vi "set_gate_parameters.vi"(4 "repetitions":i64, 5 "pulse duration (iterations)":i64, 6 "offset duration (iterations)":i64, 7 "gate no.":i32, 8 "error in (no error)":errorcluster, 9 "low phase duration (iterations)":i64, 10 "high phase duration (iterations)":i64, 11 "FPGA_AK101022Resonance in":refnum<class "FPGAWrapperAK101022Resonance.lvclass">) -> (0 "error out":errorcluster, 3 "FPGA_AK101022Resonance out":refnum<class "FPGAWrapperAK101022Resonance.lvclass">)   [LabVIEW 2010, in "FPGAWrapperAK101022Resonance.lvclass"]
uses:
  FPGAWrapperAK101022Resonance.lvclass
  common_typedefs/clock_parameters_cluster.ctl
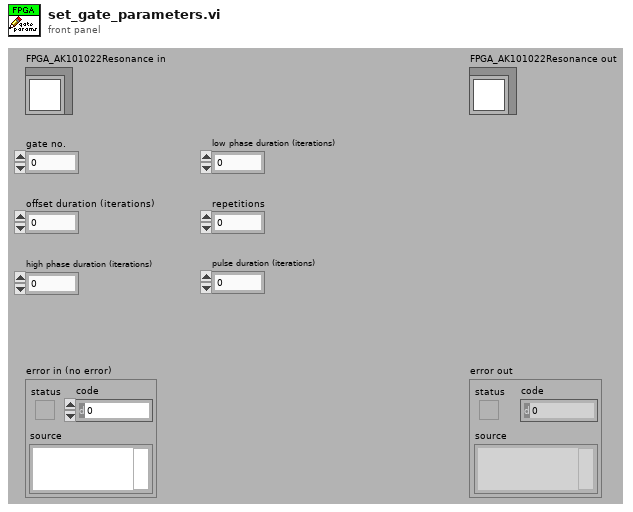
[diagram p1: front panel]
types:
  T1 = typedef "clock_parameters_cluster.ctl" = cluster{"offset":i64, "pulsing":i64, "not pulsing":i64, "cycles per pulse":i64, "repetitions":i64}
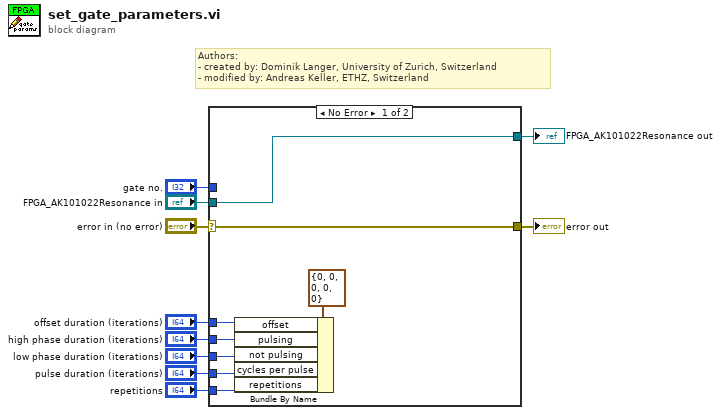
[diagram p0: block diagram]
diagram:
  # "Authors: \n- created by: Dominik Langer, University of Zurich, Switzerland\n- modified by: Andreas Keller, ETHZ, Switzerland"
  n1 = case shown="No Error" "error in (no error)" {
    selector: "error in (no error)" -> [w12 w20]
    tunnel: [w12 w20] -> w3
    tunnel: "FPGA_AK101022Resonance in" -> [w11 w19]
    tunnel: "offset duration (iterations)" -> [w17 _]
    tunnel: "high phase duration (iterations)" -> [w16 _]
    tunnel: "low phase duration (iterations)" -> [w15 _]
    tunnel: "pulse duration (iterations)" -> [w14 _]
    tunnel: "repetitions" -> [w13 _]
    tunnel: [w11 w19] -> w2
    tunnel: "gate no." -> [_ _]
    frame No Error {
      n2 = Bundle By Name(cluster=T1 {"offset"=0, "pulsing"=0, "not pulsing"=0, "cycles per pulse"=0, "repetitions"=0} ("gate settings"), "offset"=w17, "pulsing"=w16, "not pulsing"=w15, "cycles per pulse"=w14, "repetitions"=w13) -> ()  [unwired: 1 out]
    }
    frame Error {
    }
  }
  "error out" <- w3
  "FPGA_AK101022Resonance out" <- w2
